vi "WOLA_fft.vi"(10 "data in":u32, 11 "input valid":bool) -> (1 "data index":u16, 2 "output valid":bool, 3 "fft_output":u64, 4 "new fft cycle":bool)   [LabVIEW 2021]
uses:
  <vilib>/rvi/Analysis/measure/FFT/simModelSupport/niFPGA FFT Streaming Sim Properties.ctl
  <vilib>/rvi/Analysis/measure/FFT/simModelSupport/niFPGA FFT Sim Stream Group Properties.ctl
  <vilib>/rvi/Analysis/measure/FFT/simModelSupport/niFPGA FFT Sim Types.ctl
  <vilib>/rvi/Analysis/measure/FFT/simModelSupport/niFpgaFFTSimArithmeticProperties.ctl
  <vilib>/rvi/Analysis/measure/FFT/simModelSupport/niFpgaFFTSimDfxp.ctl
  <vilib>/fxp/LVFixedPointQuantizationPolicyTypeDef.ctl
  <vilib>/rvi/Analysis/measure/FFT/XNode/niFpgaFFTButterflyDelays.ctl
  <vilib>/rvi/Analysis/measure/FFT/simModelSupport/niFpgaFFTSimModelStreamingCore.vi
  <vilib>/rvi/Analysis/measure/FFT/XNode/niFpgaFFT.xnode
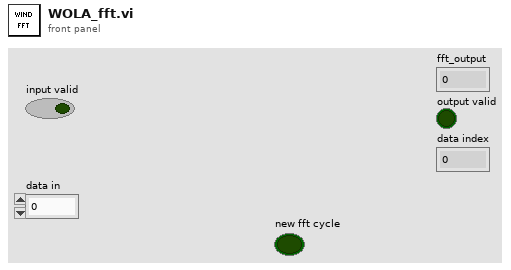
[diagram p1: front panel]
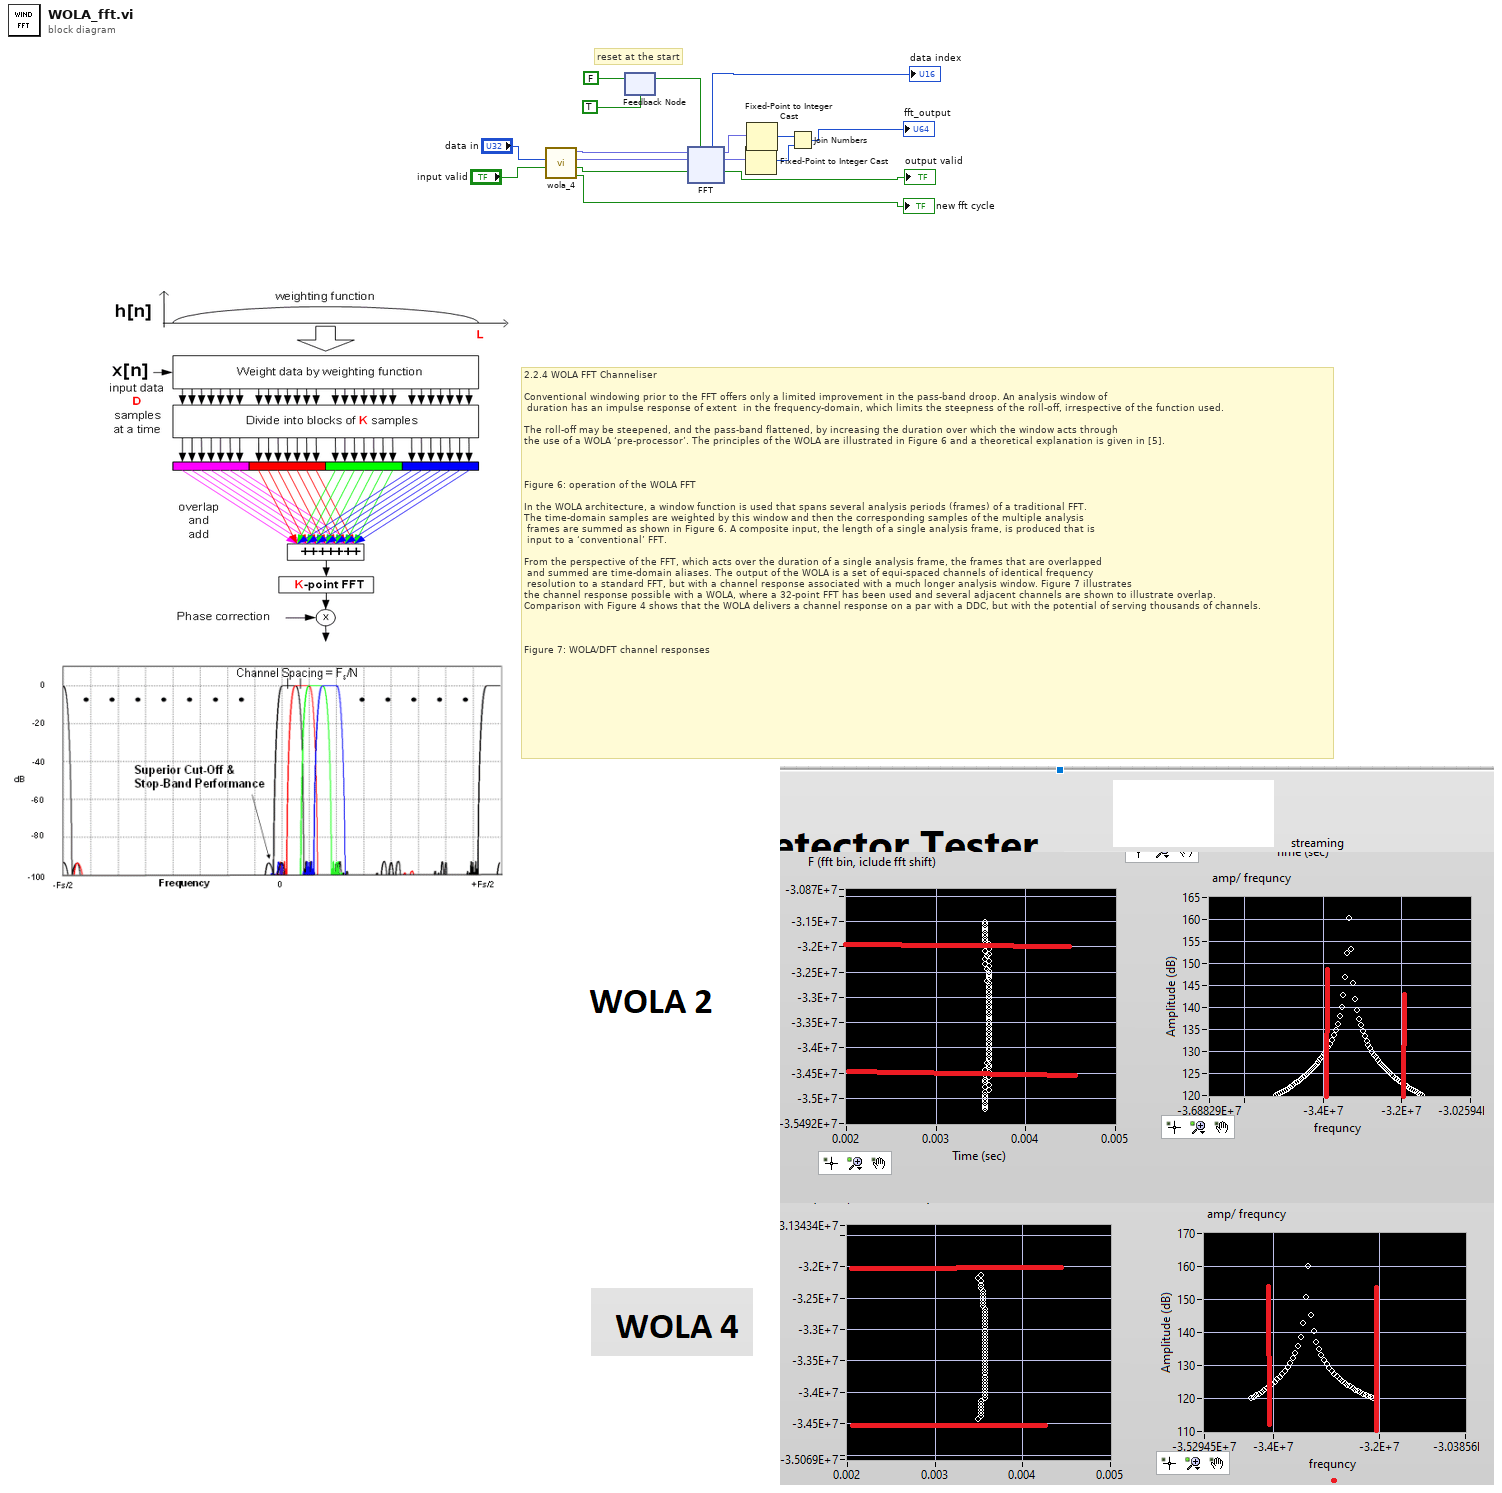
[diagram p0: block diagram]
diagram:
  # "reset at the start"
  # "2.2.4 WOLA FFT Channeliser\n\nConventional windowing prior to the FFT offers only a limited improvement in the pass-band droop. An analysis window of\n duration has an impulse response of extent  in the frequency-domain, which limits the steepness of the roll-off, irrespective of the function used.\n\nThe roll-off may be steepened, and the pass-band flattened, by increasing the duration over which the window acts through \nthe use of a WOLA ‘pre-processor’. The principles of the WOLA are illustrated in Figure 6 and a theoretical explanation is given in [5].\n\n\n\nFigure 6: operation of the WOLA FFT\n\nIn the WOLA architecture, a window function is used that spans several analysis periods (frames) of a traditional FFT. \nThe time-domain samples are weighted by this window and then the corresponding samples of the multiple analysis\n frames are summed as shown in Figure 6. A composite input, the length of a single analysis frame, is produced that is\n input to a ‘conventional’ FFT.\n\nFrom the perspective of the FFT, which acts over the duration of a single analysis frame, the frames that are overlapped\n and summed are time-domain aliases. The output of the WOLA is a set of equi-spaced channels of identical frequency\n resolution to a standard FFT, but with a channel response associated with a much longer analysis window. Figure 7 illustrates \nthe channel response possible with a WOLA, where a 32-point FFT has been used and several adjacent channels are shown to illustrate overlap. \nComparison with Figure 4 shows that the WOLA delivers a channel response on a par with a DDC, but with the potential of serving thousands of channels.\n\n\n\nFigure 7: WOLA/DFT channel responses"
  n1 = call "wola_4.vi"("input valid"="input valid", "data in"="data in") -> ("new fft loop"=→"new fft cycle":bool, "output valid"=w6:bool, "Q"=w5:fxp<+/-,21,18>, "I"=w4:fxp<+/-,21,18>)  [unwired: 6 in]
  n2 = feedback #1(TRUE ("use zero instead of x")) -> (w9:bool)
  n3 = feedback-in #1(FALSE ("use zero instead of x")) -> ()
  n4 = xnode ("FFT")("real data in"=w4, "reset"=w9, "imaginary data in"=w5, "input valid"=w6) -> ("data index"=→"data index":u16, "real data out"=w12:fxp<+/-,32,31>, "imaginary data out"=w13:fxp<+/-,32,31>, "output valid"=→"output valid":bool)  [unwired: 1 in, 1 out]
  n5 = Fixed-Point to Integer Cast(1:w13) -> (0:w15:i32)
  n6 = Fixed-Point to Integer Cast(1:w12) -> (0:w14:i32)
  n7 = Join Numbers(hi=w14, lo=w15) -> ((hi.lo)=→"fft_output":u64)
